vi "fgv_Sweep_chirp_compute_ref.vi"(7 "FGV Actions":T1, 8 "error in (no error)":errorcluster) -> (0 "error out":errorcluster, 3 "VI Refnum":refnum<vi>)   [LabVIEW 2017]
uses:
  Typedefs/fgv_actions.ctl
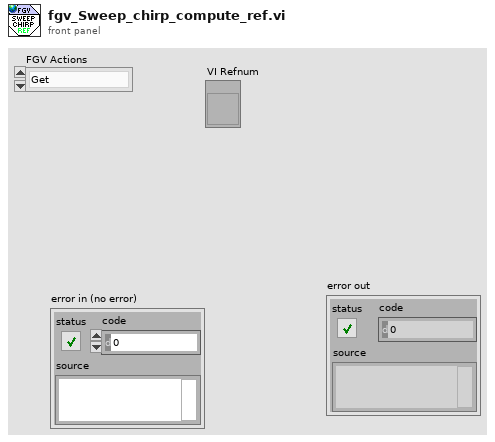
[diagram p1: front panel]
types:
  T1 = typedef "fgv_actions.ctl" = enum16{"Get", "Set"}
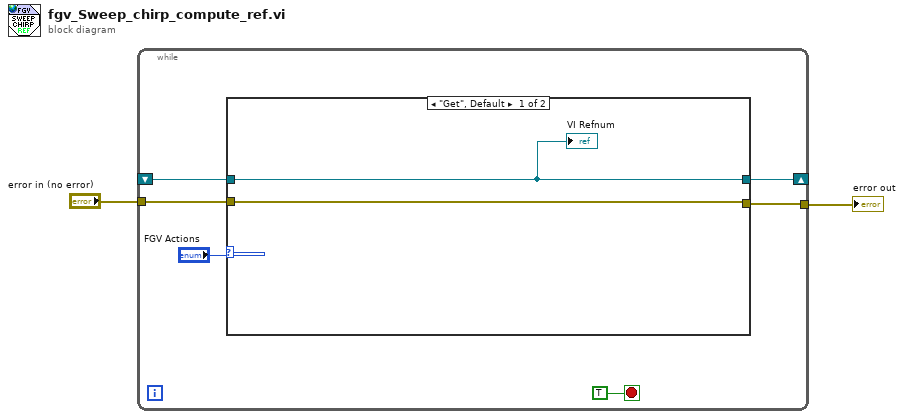
[diagram p0: block diagram]
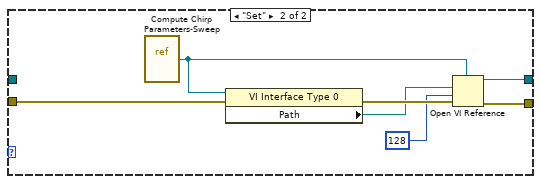
[diagram p2: hidden frame]
diagram:
  n1 = while {
    tunnel: [w5] -> w2
    tunnel: "error in (no error)" -> [w6]
    shift-right: [w4] -> _
    shift-left: _ -> [w3]
    stop <- TRUE stop-if-true
    n2 = case shown="\"Get\", Default" "FGV Actions" {
      tunnel: w6 -> [w9 w13]
      tunnel: [w9 w12] -> w5
      tunnel: [w10 w11] -> w4
      tunnel: w3 -> [w10 _]
      frame "Get", Default {
        "VI Refnum" <- w10
      }
      frame "Set" {
        n3 = vi-ref "Compute Chirp Parameters-Sweep.vi"() -> (w15:refnum<vi>)
        n4 = property class="VI Interface Type 0"(reference=w15, error in=w13) -> (error out=w17:errorcluster, "Path"=w16:path)  [unwired: 1 out]
        n5 = Open VI Reference(type specifier VI Refnum (for type only)=w15, vi path=w16, options=128, error in (no error)=w17) -> (vi reference=w11:refnum<vi>, error out=w12:errorcluster)  [unwired: 2 in]
      }
    }
  }
  "error out" <- w2
